vi "Create.vi"(8 "error in (no error)":errorcluster, 10 "Element":refnum<class "Config Element.lvclass">) -> (0 "error out":errorcluster, 3 "System out":refnum<class "System Config.lvclass">)   [LabVIEW 2020, in "VolatusConfig.lvlib" / "System Config.lvclass"]
uses:
  System Config.lvclass
  C:/dev/lv20CE/relink/lv-volatus/VolatusConfig/VolatusConfigElement/VolatusConfigElement.lvclass
  lv-cdm/CDM-Config/Config Element/Config Element.lvclass
  System Config.lvclass/System Config.ctl
  VolatusConfigElement/VolatusConfigElement.lvclass
  C:/dev/lv20CE/relink/lv-volatus/VolatusConfig/System/System Config.lvclass
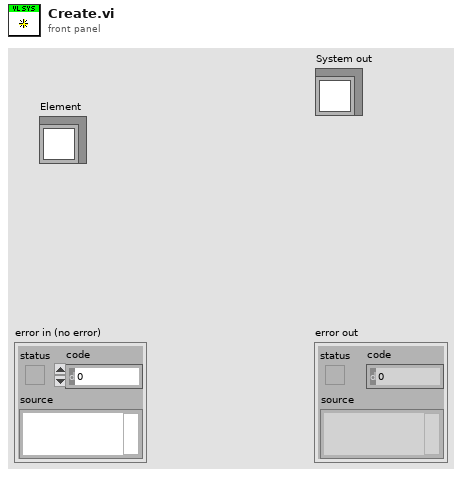
[diagram p1: front panel]
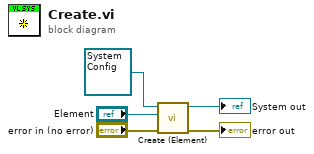
[diagram p0: block diagram]
diagram:
  n1 = call "Create (Element).vi"("error in (no error)"="error in (no error)", "Element"="Element", "VolatusConfigElement in"=refnum<class "System Config.lvclass"> refnum ("System in")) -> ("error out"=→"error out":errorcluster, "VolatusConfigElement out"=→"System out":refnum<class "System Config.lvclass">)  [unwired: 7 in]
